vi "Append Phrase.vi"(0 "PDF Report IN":refnum<class "PDF Report Class.lvclass">, 2 "Text":string, 11 "error in (no error)":errorcluster, 12 "Font":T2={"Name"="", "Size"=-1.0, "Color"=0, "Style"={"Bold"=FALSE, "Italic"=FALSE, "Underline"=FALSE, "Strikeout"=FALSE}, "Type"={"Type&direction"=enum."Select", "Embedded"=FALSE, "Encoding"=""}}, 14 "Line spacing":T1) -> (4 "PDF Report OUT":refnum<class "PDF Report Class.lvclass">, 15 "error out":errorcluster)   [LabVIEW 2020, in "Exaprom PDF.lvlib"]
doc: "Appends text to the PDF report. This text <B>can not</B> be aligned and indented. \n\nIf <B>Font</B> is not specified then the <B>Default font</B> will be use.\n\nThe data type you wire to the <B>Text</B> input determines the polymorphic instance to use.\n\n<B>FRANÇAIS</B>\nAjoute du texte au rapport. Ce texte ne peut être <B>aligné</B> et ne peut avoir un <B>renfoncement</B>.\n\nSi la police de caractères <B>Font</B> n'est pas spécifiée alors la <B>police de caractères par défaut</B> sera utilisée.\n\nLe type de données que vous connectez au terminal <B>Text</B> détermine l'instance polymorphique utilisée.\nVersion 2.0\nDeveloped by Jean-Marc Simard\nCopyright © 2012, Exaprom Inc.\nAll rights reserved.\nLicense: BSD\n\nWith iTextSharp 4.1.6 (http://itextsharp.sourceforge.net)\nunder Mozilla Public License Version 1.1\n(http://www.mozilla.org/MPL/MPL-1.1.html)"
uses:
  <userlib>/labview-PDF-writer-master/Exaprom PDF.lvlib
  <userlib>/labview-PDF-writer-master/Controls/Font Controls/Font complete cluster.ctl
  <userlib>/labview-PDF-writer-master/Controls/Font Controls/Font size.ctl
  <userlib>/labview-PDF-writer-master/Controls/Font Controls/Font color.ctl
  <userlib>/labview-PDF-writer-master/Controls/Font Controls/Type and encoding.ctl
  <userlib>/labview-PDF-writer-master/Controls/Text Controls/Unicode/Type and run direction.ctl
  <userlib>/labview-PDF-writer-master/LV Class/PDF Report Class/PDF Report Class.lvclass
  <userlib>/labview-PDF-writer-master/Controls/Text Controls/Line spacing.ctl
  <userlib>/labview-PDF-writer-master/Controls/Text Controls/Texte alignement.ctl
  C:/Program Files (x86)/National Instruments/LabVIEW 2020/user.lib/labview-PDF-writer-master/DLL/itextsharp.dll
  DLL/itextsharp.dll
  <userlib>/labview-PDF-writer-master/LV Class/Fonts Class/Font Class.lvclass
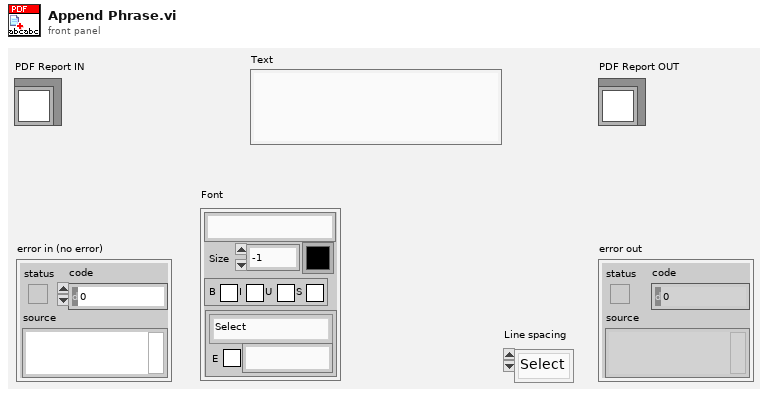
[diagram p1: front panel]
types:
  T1 = typedef "Exaprom PDF.lvlib/Line spacing.ctl" = enum16{"Select", "1.0", "1.5", "2.0"}
  T2 = typedef "Exaprom PDF.lvlib/Font complete cluster.ctl" = cluster{"Name":string, "Size":T3, "Color":T4, "Style":cluster{"Bold":bool, "Italic":bool, "Underline":bool, "Strikeout":bool}, "Type":T5}
  T3 = typedef "Exaprom PDF.lvlib/Font size.ctl" = sgl
  T4 = typedef "Exaprom PDF.lvlib/Font color.ctl" = u32
  T5 = typedef "Exaprom PDF.lvlib/Type and encoding.ctl" = cluster{"Type&direction":T6, "Embedded":bool, "Encoding":string}
  T6 = typedef "Exaprom PDF.lvlib/Type and run direction.ctl" = enum16{"Select", "ASCII", "UTF-16", "UTF-16 (default)", "UTF-16 (LTR)", "UTF-16 (RTL)"}
  T7 = typedef "Exaprom PDF.lvlib/Texte alignement.ctl" = enum16{"Select", "CENTER", "JUSTIFY", "LEFT", "RIGHT"}
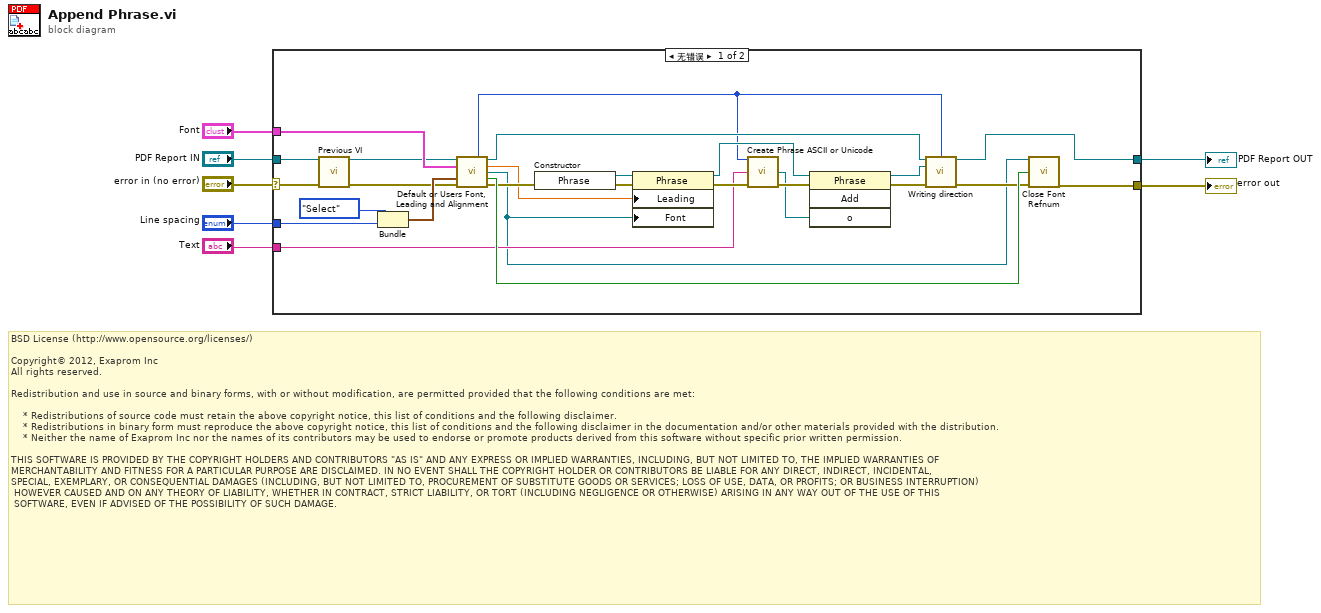
[diagram p0: block diagram]
diagram:
  # "BSD License (http://www.opensource.org/licenses/)\n\nCopyright© 2012, Exaprom Inc\nAll rights reserved.\n\nRedistribution and use in source and binary forms, with or without modification, are permitted provided that the following conditions are met:\n\n    * Redistributions of source code must retain the above copyright notice, this list of conditions and the following disclaimer.\n    * Redistributions in binary form must reproduce the above copyright notice, this list of conditions and the following disclaimer in the documentation and/or other materials provided with the distribution.\n    * Neither the name of Exaprom Inc nor the names of its contributors may be used to endorse or promote products derived from this software without specific prior written permission.\n\nTHIS SOFTWARE IS PROVIDED BY THE COPYRIGHT HOLDERS AND CONTRIBUTORS \"AS IS\" AND ANY EXPRESS OR IMPLIED WARRANTIES, INCLUDING, BUT NOT LIMITED TO, THE IMPLIED WARRANTIES OF \nMERCHANTABILITY AND FITNESS FOR A PARTICULAR PURPOSE ARE DISCLAIMED. IN NO EVENT SHALL THE COPYRIGHT HOLDER OR CONTRIBUTORS BE LIABLE FOR ANY DIRECT, INDIRECT, INCIDENTAL,\nSPECIAL, EXEMPLARY, OR CONSEQUENTIAL DAMAGES (INCLUDING, BUT NOT LIMITED TO, PROCUREMENT OF SUBSTITUTE GOODS OR SERVICES; LOSS OF USE, DATA, OR PROFITS; OR BUSINESS INTERRUPTION)\n HOWEVER CAUSED AND ON ANY THEORY OF LIABILITY, WHETHER IN CONTRACT, STRICT LIABILITY, OR TORT (INCLUDING NEGLIGENCE OR OTHERWISE) ARISING IN ANY WAY OUT OF THE USE OF THIS\n SOFTWARE, EVEN IF ADVISED OF THE POSSIBILITY OF SUCH DAMAGE."
  n1 = case shown="无错误" "error in (no error)" {
    selector: "error in (no error)" -> [w33 w35]
    tunnel: "Font" -> [w11 _]
    tunnel: [w13 w34] -> w1
    tunnel: [w27 w35] -> w2
    tunnel: "PDF Report IN" -> [w32 w34]
    tunnel: "Line spacing" -> [w31 _]
    tunnel: "Text" -> [w21 _]
    frame No Error {
      n2 = call <userlib>:"Previous VI.vi"("PDF Report IN"=w32, "error in (no error)"=w33) -> ("PDF Report OUT"=w8:refnum<class "PDF Report Class.lvclass">, "error out"=w9:errorcluster)  [unwired: 12 out]
      n3 = Bundle("Aligment"=Texte_alignement."Select", "Line spacing"=w31) -> (w30:cluster{"Aligment":T7, "Line spacing":T1})  [unwired: 1 out]
      n4 = call <userlib>:"Default or Users Font, Leading and Alignment.vi"("PDF Report"=w8, "Font"=w11, "Paragraphe cluster"=w30, "error in (no error)"=w9) -> ("Type and run direction"=w10:T6, "PDF Report duplicate"=w15:refnum<class "PDF Report Class.lvclass">, "Leading"=w23:T3, "Font Ref"=w12:refnum<k24>, "Close Font Ref"=w28:bool, "error out"=w24:errorcluster)  [unwired: 6 out]
      n5 = constructor class="Phrase"(error in=w24) -> (reference out=w25:refnum<k24>, error out=w26:errorcluster)  [unwired: 2 in, 1 out]
      n6 = property class="Phrase"(reference=w25, error in=w26, "Leading"=w23, "Font"=w12) -> (reference out=w19:refnum<k24>, error out=w22:errorcluster)
      n7 = call <userlib>:"Create Phrase ASCII or Unicode.vi"("Character type"=w10, "Text"=w21, "error in (no error)"=w22) -> ("Phrase refnum"=w18:refnum<k24>, "error out"=w20:errorcluster)  [unwired: 10 in, 1 out]
      n8 = invoke class="Phrase" method="Add"(reference=w19, error in=w20, "o"=w18) -> (reference out=w16:refnum<k24>, error out=w17:errorcluster)  [unwired: 1 in, 2 out]
      n9 = call <userlib>:"Writing direction.vi"("PDF Report IN"=w15, "Text type"=w10, "Phrase refnum"=w16, "error in (no error)"=w17) -> ("PDF Report OUT"=w13:refnum<class "PDF Report Class.lvclass">, "error out"=w14:errorcluster)  [unwired: 10 in]
      n10 = call <userlib>:"Close Font Refnum.vi"("Font Refnum"=w12, "Close ?"=w28, "error in (no error)"=w14) -> ("error out"=w27:errorcluster)  [unwired: 12 in]
    }
    frame Error {
    }
  }
  "PDF Report OUT" <- w1
  "error out" <- w2
